vi "Get Experiment Information.vi"(8 "error in (no error)":errorcluster, 10 "devices off":string[](array[string]), 11 "> Expt Name >":string) -> (0 "error out":errorcluster, 1 "> UDP cluster for Shot ctrl Dev >":T2, 2 "> devices to get data from during scan >":string[](array[string]), 3 "> Name of Shot dev >":string, 4 "> Subscribtion variables with devices  for Scan >":string[](array[string]), 5 "> Scan data to get (from Expt editor)>":string[][](array[string]), 6 "expt devices":string[](array[string]), 7 "scans path":path, 9 "TCP subscriptions info":T1)   [LabVIEW 2020]
uses:
  UDP send cluster.ctl
  Shared/GUI_Template/TCP subscription info cluster.ctl
  Shared/MySQL/Preset Query Enum.ctl
  <userlib>/_OpenG.lib/array/array.llb/Search 1D Array (String)__ogtk.vi
  <userlib>/_OpenG.lib/array/array.llb/Delete Elements from 2D Array (String)__ogtk.vi
panel:
  out "subarray":string[](array[string])
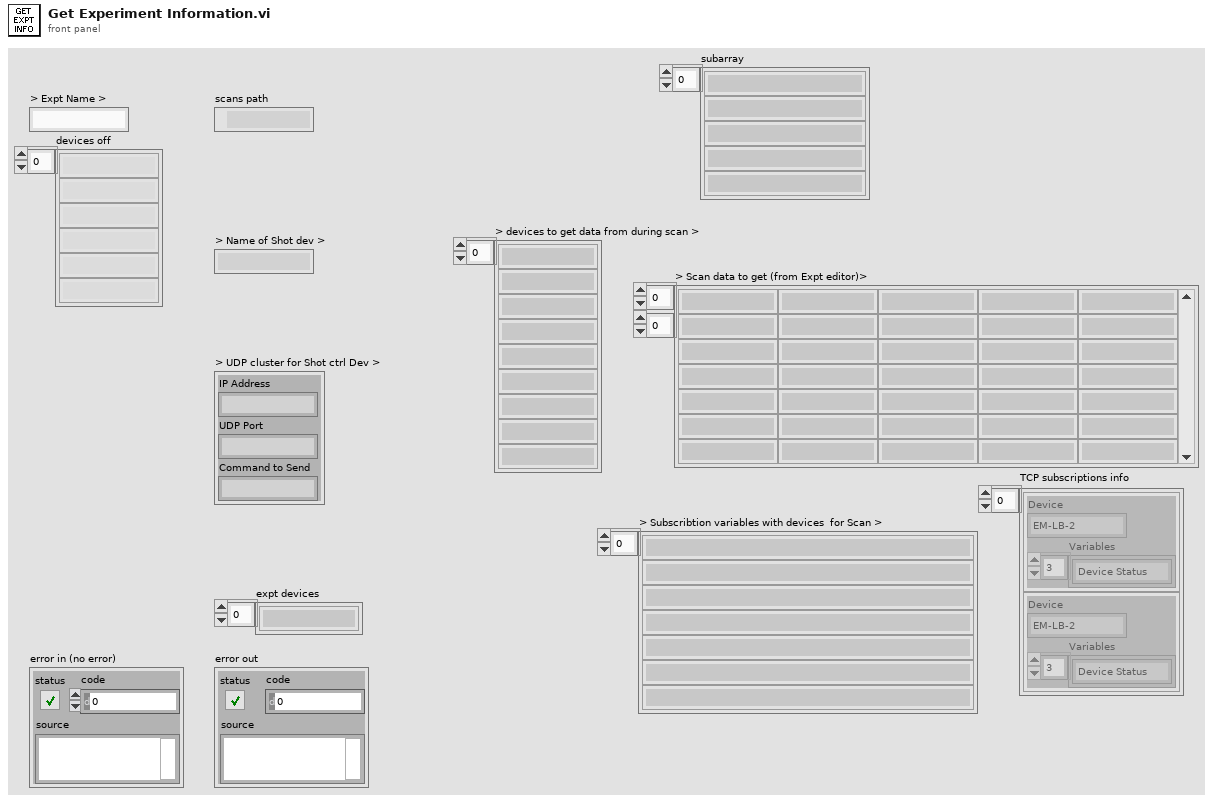
[diagram p1: front panel]
types:
  T1 = typedef "TCP subscription info cluster.ctl" = cluster{"Device":string, "Variables":string[]}[]
  T2 = typedef "UDP send cluster.ctl" = cluster{"IP Address":string, "UDP Port":string, "Command to Send":string}
  T3 = typedef "Preset Query Enum.ctl" = enum16{"Get Locations", "Get all IPs and MACs", "Get classes", "Get expt variables to set at scanstart for particular device", "Get expt devices and variables with start values", "Get expt devices and variables (with data to get)", "Get expt devices with data to get", "Get Expt devices and GUIs", "Get all devices basic properties", "Get Virtual Devices Core Info", "Get Expt names", "Get experiment basic properties", "Get experiment alarm variables", "Get MC Ports", "Get device network comm port", "Get devicetype lvclass path", "Get basic device properties", "Get Init Order", "Get all setable variables of a device", "Get device variable aliases", "Get force values of all settable variables", "Get all variables of a devicetype", "Get all variables of a device", "Get plotter details", "Get Saved Scans", "Get Scan Info", "GetGeneralGUIs", "Get expt for plotter", "Get plotter IDs from expt", "Get all devices", "Get all Virtual Devices", "Get all aliases", "Get variable and device info for Virtual Device", "GetItemLocatorIP", "Get IPs for GUIs", "Get DeviceType from Device", "GetLocalPortRange", "GetDevicePresetVariables", "Get Device Configuration", "GetAllPresetNames", "GetAllConfigurationNames", "GetPresetDeviceNames", "GetDeviceAliases", "GetDevicesOfClass"}
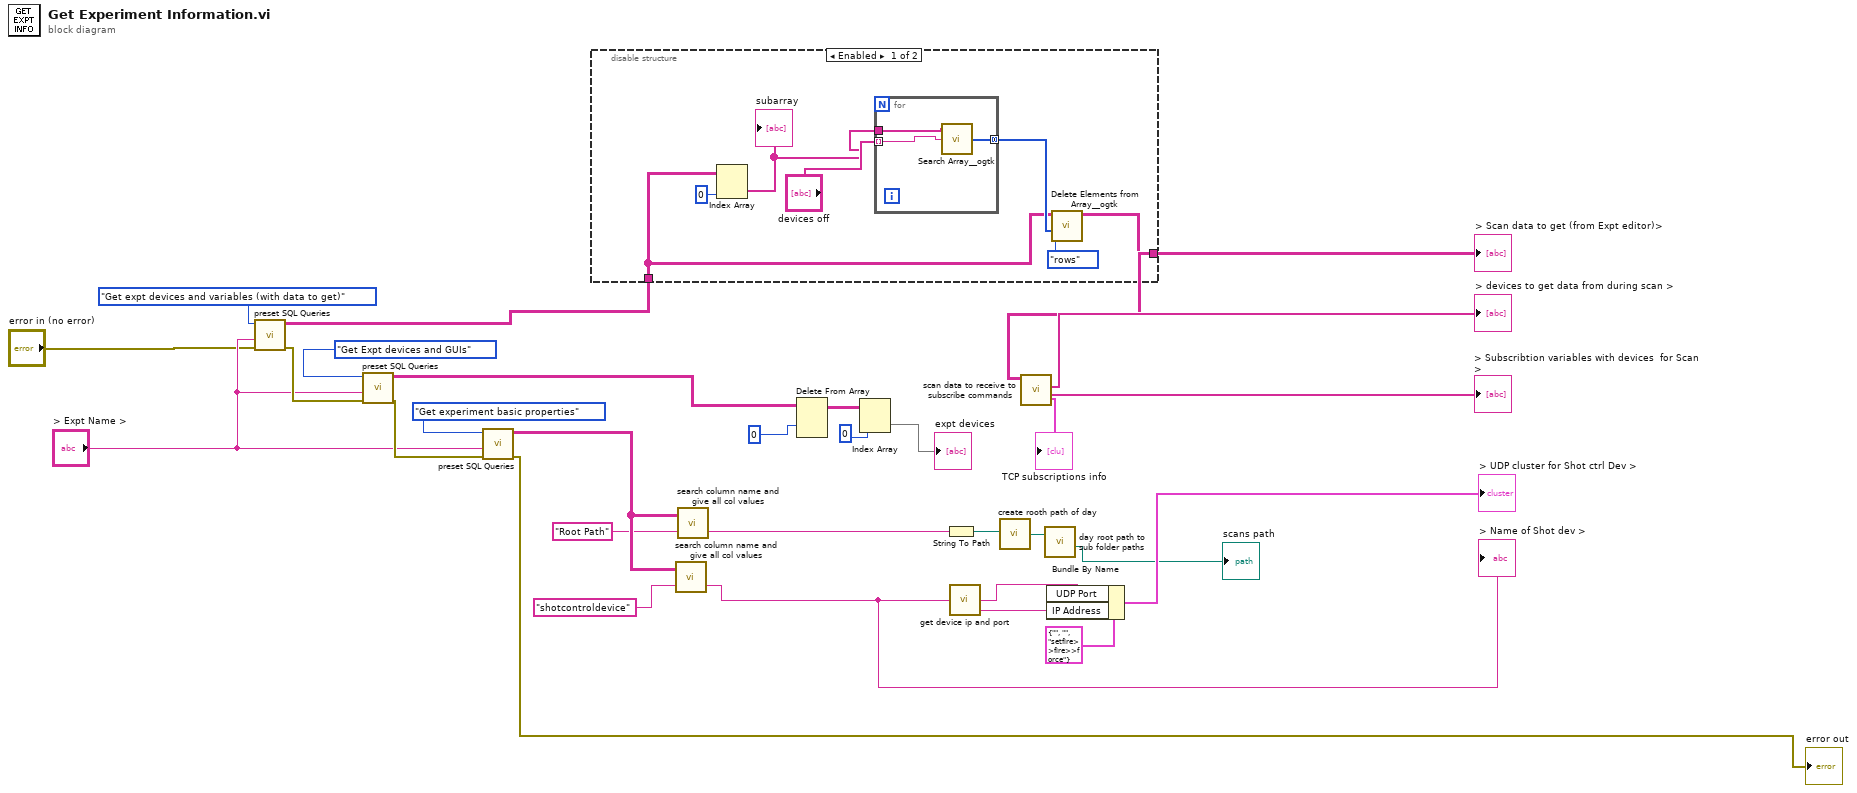
[diagram p0: block diagram]
diagram:
  n1 = call "preset SQL Queries.vi"("error in (no error)"="error in (no error)", "Expt name / MCIP/ Variable/Preset Name"="> Expt Name >", "Preset Query"=Preset_Query_Enum."Get expt devices and variables (with data to get)") -> ("error out"=w16:errorcluster, "data"=w2:string[][])  [unwired: 6 in, 1 out]
  n2 = call "preset SQL Queries.vi"("error in (no error)"=w16, "Expt name / MCIP/ Variable/Preset Name"="> Expt Name >", "Preset Query"=Preset_Query_Enum."Get Expt devices and GUIs") -> ("error out"=w22:errorcluster, "data"=w7:string[][])  [unwired: 6 in, 1 out]
  n3 = call "preset SQL Queries.vi"("error in (no error)"=w22, "Expt name / MCIP/ Variable/Preset Name"="> Expt Name >", "Preset Query"=Preset_Query_Enum."Get experiment basic properties") -> ("error out"=→"error out":errorcluster, "data"=w30:string[][])  [unwired: 6 in, 1 out]
  n4 = disable-structure shown="Enabled" {
    disable-tunnel: w2 -> [w33 w41]
    disable-tunnel: [w32 w41] -> w1
    frame Enabled {
      n5 = Index Array(array=w33, index (col)=0 ("disabled index (col)")) -> (element=w34:string[])  [unwired: 1 in]
      "subarray" <- w34
      n6 = for {
        tunnel: "devices off" -> [w39] mode=indexing
        tunnel: w34 -> [w40]
        tunnel: [w38] -> w36 mode=concatenating
        n7 = call-poly <userlib>:"Search Array__ogtk.vi"("Array"=w40, "Element Data"=w39) -> ("Indices of Elements"=w38:i32[])  [unwired: 7 in]
      }
      n8 = call-poly <userlib>:"Delete Elements from Array__ogtk.vi"("delete (rows or columns)"=enum16{"rows", "columns"}."rows", "indices"=w36, "array"=w33) -> ("array w/ subset deleted"=w32:string[][])  [unwired: 7 in, 1 out]
    }
    frame Disabled {
    }
  }
  "> Scan data to get (from Expt editor)>" <- w1
  n9 = call "search column name and give all col values.vi"("column name to get"="shotcontroldevice", "input 2d array"=w30) -> ("First value"=w28:string)  [unwired: 1 out]
  "> Name of Shot dev >" <- w28
  n10 = call "search column name and give all col values.vi"("column name to get"="Root Path", "input 2d array"=w30) -> ("First value"=w17:string)  [unwired: 1 out]
  n11 = Delete From Array(array=w7, index (row)=0) -> (array with subset deleted=w5:string[][])  [unwired: 2 in, 1 out]
  n12 = Index Array(array=w5, index (col)=0 ("disabled index (col)")) -> (element=→"expt devices":string[])  [unwired: 1 in]
  n13 = String To Path(string=w17) -> (path=w19:path)
  n14 = call "get device ip and port.vi"("variable1"=w28) -> ("port"=w26:string, "IP"=w25:string)  [unwired: 1 out]
  n15 = call "create rooth path of day.vi"("Expt root path"=w19) -> ("Day path"=w18:path)
  n16 = call "scan data to receive to subscribe commands.vi"("ScanData to receive"=w1) -> ("dev space var"=→"> Subscribtion variables with devices  for Scan >":string[], "devices"=→"> devices to get data from during scan >":string[], "TCP subscriptions info"=→"TCP subscriptions info":T1)  [unwired: 7 in, 1 out]
  n17 = call "day root path to sub folder paths.vi"("day root path"=w18) -> ("scans path"=→"scans path":path)  [unwired: 4 out]
  n18 = Bundle By Name(cluster=T2 {"IP Address"="", "UDP Port"="", "Command to Send"="setfire>>fire>>force"} ("UDP Send Cluster"), "UDP Port"=w26, "IP Address"=w25) -> (→"> UDP cluster for Shot ctrl Dev >":T2)
